vi "SetAttr Enum.vi"(8 "error in (no error)":errorcluster, 9 "EnumU32Value":u32, 10 "AttributeName":string, 11 "IMAQdx Actor in":refnum<class "IMAQdx Actor.lvclass">) -> (0 "error out":errorcluster, 3 "IMAQdx Actor out":refnum<class "IMAQdx Actor.lvclass">)   [LabVIEW 2020, in "IMAQdx Actor.lvlib" / "IMAQdx Actor.lvclass"]
uses:
  IMAQdx Actor.lvclass
  IMAQdx Actor.lvclass/IMAQdx Actor.ctl
  <resource>/objmgr/imaqdx.rc
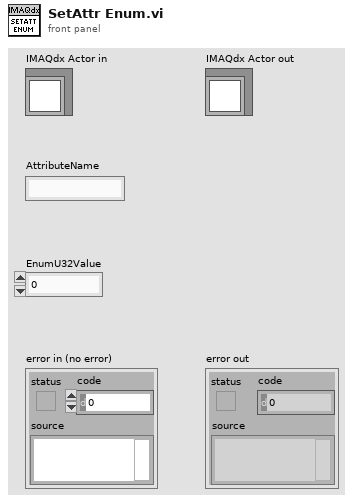
[diagram p1: front panel]
types:
  T1 = typedef "IMAQdx.ctl" = refnum<k21>
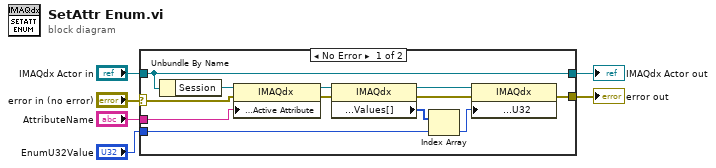
[diagram p0: block diagram]
diagram:
  n1 = case shown="No Error" "error in (no error)" {
    selector: "error in (no error)" -> [w8 w20]
    tunnel: [w7 w20] -> w5
    tunnel: [w18 w19] -> w3
    tunnel: "IMAQdx Actor in" -> [w18 w19]
    tunnel: "AttributeName" -> [w16 _]
    tunnel: "EnumU32Value" -> [w11 _]
    frame No Error {
      n2 = Unbundle By Name(w18) -> ("Session"=w17:T1)
      n3 = property class="IMAQdx"(reference=w17, error in=w8, "Camera Attributes:Active Attribute"=w16) -> (reference out=w10:T1, error out=w9:errorcluster)
      n4 = property class="IMAQdx"(reference=w10, error in=w9) -> (reference out=w12:T1, error out=w13:errorcluster, "Camera Attributes:Enum:Values[]"=w14:u32[])
      n5 = Index Array(array=w14, index=w11) -> (element=w15:u32)
      n6 = property class="IMAQdx"(reference=w12, error in=w13, "Camera Attributes:Value:U32"=w15) -> (error out=w7:errorcluster)  [unwired: 1 out]
    }
    frame Error {
    }
  }
  "error out" <- w5
  "IMAQdx Actor out" <- w3
